vi "ManipulaData.vi"(10 "Error en fechas?":bool, 11 "Data In":string[][](array[string])) -> (3 "Historico Out":cluster{dbl[], dbl[]}[](array[cluster]), 5 "Data a exportar":dbl[][](array[numeric]))   [LabVIEW 2018]
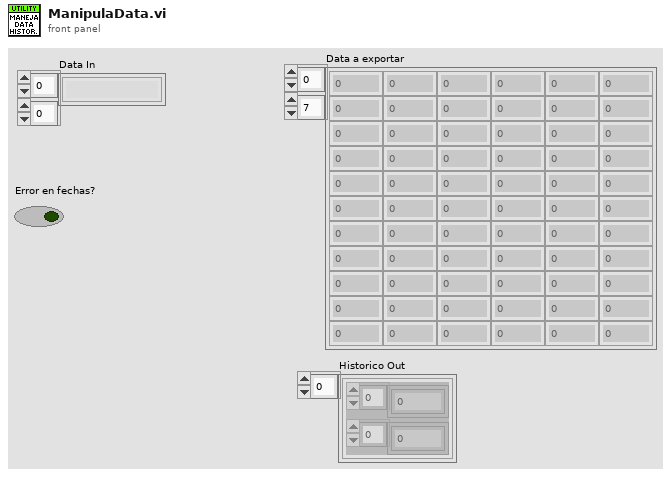
[diagram p1: front panel]
types:
  T1 = typedef "LVDateTimeRec.ctl" = cluster{"fractional second":dbl, "second":i32, "minute":i32, "hour":i32, "day of month":i32, "month":i32, "year":i32, "day of week":i32, "day of year":i32, "DST":i32}
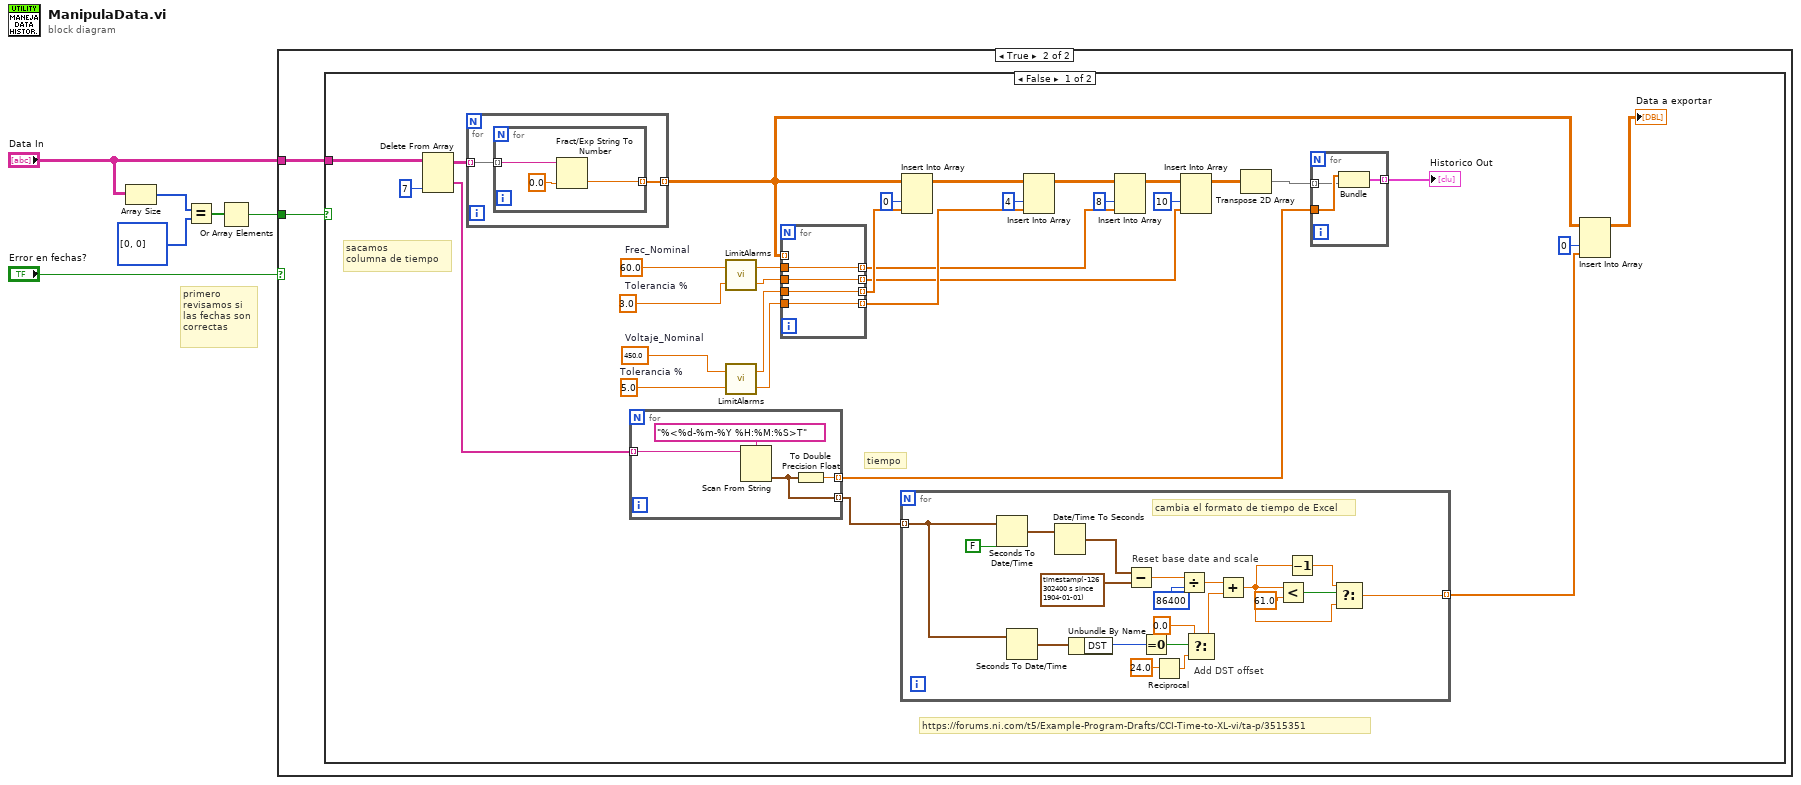
[diagram p0: block diagram]
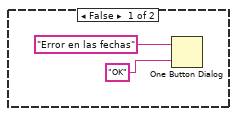
[diagram p2: hidden frame]
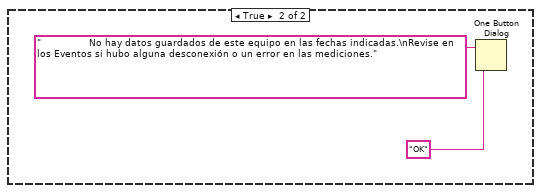
[diagram p3: hidden frame]
diagram:
  # "primero \nrevisamos si \nlas fechas son\ncorrectas"
  n1 = Array Size(array="Data In") -> (size(s)=w6:i32[])
  n2 = Equal?(x=w6, y=i32[] [0, 0] ("size(s)")) -> (x = y?=w4:bool[])
  n3 = Or Array Elements(Boolean array=w4) -> (logical OR=w3:bool)
  n4 = case shown="True" "Error en fechas?" {
    tunnel: w3 -> [_ w10]
    tunnel: "Data In" -> [_ w9]
    frame False {
      n5 = One Button Dialog(message="Error en las fechas", button name ("OK")="OK") -> ()  [unwired: 1 out]
    }
    frame True {
      n6 = case shown="False" w10 {
        tunnel: w9 -> [w17 _]
        frame False {
          w39 = sgl 5.0  # Tolerancia %
          w40 = sgl 450.0  # Voltaje_Nominal
          w35 = sgl 3.0  # Tolerancia %
          w36 = sgl 60.0  # Frec_Nominal
          # "https://forums.ni.com/t5/Example-Program-Drafts/CCI-Time-to-XL-vi/ta-p/3515351"
          # "tiempo"
          # "sacamos \ncolumna de tiempo"
          n7 = Delete From Array(array=w17, index (col)=7 ("disabled index (col)")) -> (deleted portion=w34:string[], array with subset deleted=w33:string[][])  [unwired: 2 in]
          n8 = for {
            tunnel: w33 -> [w75] mode=indexing
            tunnel: [w74] -> w16 mode=indexing
            n9 = for {
              tunnel: w75 -> [w76] mode=indexing
              tunnel: [w77] -> w74 mode=indexing
              n10 = Fract/Exp String To Number(string=w76, default (0 dbl)=0.0 ("default (0 DBL)")) -> (number=w77:dbl)  [unwired: 2 in, 1 out]
            }
          }
          n11 = for {
            tunnel: w34 -> [w70] mode=indexing
            tunnel: [w72] -> w14 mode=indexing
            tunnel: [w71] -> w12 mode=indexing
            n12 = Scan From String(format string="%<%d-%m-%Y %H:%M:%S>T", input string=w70) -> (output 1=w71:timestamp)  [unwired: 3 in, 3 out]
            n13 = To Double Precision Float(number=w71) -> (double precision float=w72:dbl)
          }
          n14 = call "LimitAlarms.vi"("Value"=w35, "Parameter"=w36) -> ("Min"=w38:sgl, "Max"=w37:sgl)
          n15 = call "LimitAlarms.vi"("Value"=w39, "Parameter"=w40) -> ("Min"=w42:sgl, "Max"=w41:sgl)
          n16 = for {
            tunnel: [w66] -> w23 mode=indexing
            tunnel: w16 -> [_] mode=indexing
            tunnel: [w65] -> w20 mode=indexing
            tunnel: w37 -> [w66]
            tunnel: w38 -> [w65]
            tunnel: [w64] -> w29 mode=indexing
            tunnel: w41 -> [w64]
            tunnel: [w63] -> w26 mode=indexing
            tunnel: w42 -> [w63]
          }
          n17 = for {
            tunnel: w12 -> [w44] mode=indexing
            tunnel: [w43] -> w11 mode=indexing
            # "cambia el formato de tiempo de Excel"
            # "Add DST offset"
            # "Reset base date and scale"
            n18 = Seconds To Date/Time(time stamp (now)=w44, to UTC (F)=FALSE ("is UTC (F)")) -> (date time rec=w58:T1)
            n19 = Seconds To Date/Time(time stamp (now)=w44) -> (date time rec=w57:T1)  [unwired: 1 out]
            n20 = Date/Time To Seconds(2:w58) -> (0:w61:timestamp)  [unwired: 1 out]
            n21 = Unbundle By Name(w57) -> ("DST"=w56:i32)
            n22 = Subtract(x=w61, y=timestamp(-126302400 s since 1904-01-01) ("time stamp 2")) -> (x-y=w60:dbl)
            n23 = Equal To 0?(x=w56) -> (x = 0?=w55:bool)
            n24 = Reciprocal(x=24.0 ("f")) -> (1/x=w52:dbl)
            n25 = Divide(x=w60, y=86400) -> (x/y=w50:dbl)
            n26 = Select(t=0.0, s=w55, f=w52) -> (s? t:f=w49:dbl)
            n27 = Add(x=w50, y=w49) -> (x+y=w46:dbl)
            n28 = Less?(x=w46, y=61.0) -> (x < y?=w47:bool)
            n29 = Decrement(x=w46) -> (x-1=w45:dbl)
            n30 = Select(t=w45, s=w47, f=w46) -> (s? t:f=w43:dbl)
          }
          n31 = Insert Into Array(array=w16, index (col)=0 ("disabled index (col)"), new element=w29) -> (w30:dbl[][])  [unwired: 1 in]
          n32 = Insert Into Array(array=w30, index (col)=4 ("disabled index (col)"), new element=w26) -> (w27:dbl[][])  [unwired: 1 in]
          n33 = Insert Into Array(array=w27, index (col)=8 ("disabled index (col)"), new element=w23) -> (w24:dbl[][])  [unwired: 1 in]
          n34 = Insert Into Array(array=w24, index (col)=10 ("disabled index (col)"), new element=w20) -> (w21:dbl[][])  [unwired: 1 in]
          n35 = Transpose 2D Array(2D array=w21) -> (transposed array=w31:dbl[][])
          n36 = for {
            tunnel: [w69] -> w18 mode=indexing
            tunnel: w14 -> [w68]
            tunnel: w31 -> [w67] mode=indexing
            n37 = Bundle(w68, w67) -> (w69:cluster{dbl[], dbl[]})  [unwired: 1 in]
          }
          "Historico Out" <- w18
          n38 = Insert Into Array(array=w16, index (col)=0 ("disabled index (col)"), new element=w11) -> (→"Data a exportar":dbl[][])  [unwired: 1 in]
        }
        frame True {
          n39 = One Button Dialog(message="                No hay datos guardados de este equipo en las fechas indicadas.\nRevise en los Eventos si hubo alguna desconexión o un error en las mediciones.", button name ("OK")="OK") -> ()  [unwired: 1 out]
        }
      }
    }
  }
